vi "James_LED.vi"   [LabVIEW 2023]
uses:
  <vilib>/Rock Robotics/WPI/ThirdParty/PhotonVisionLib/PhotonVisionLib.lvlib
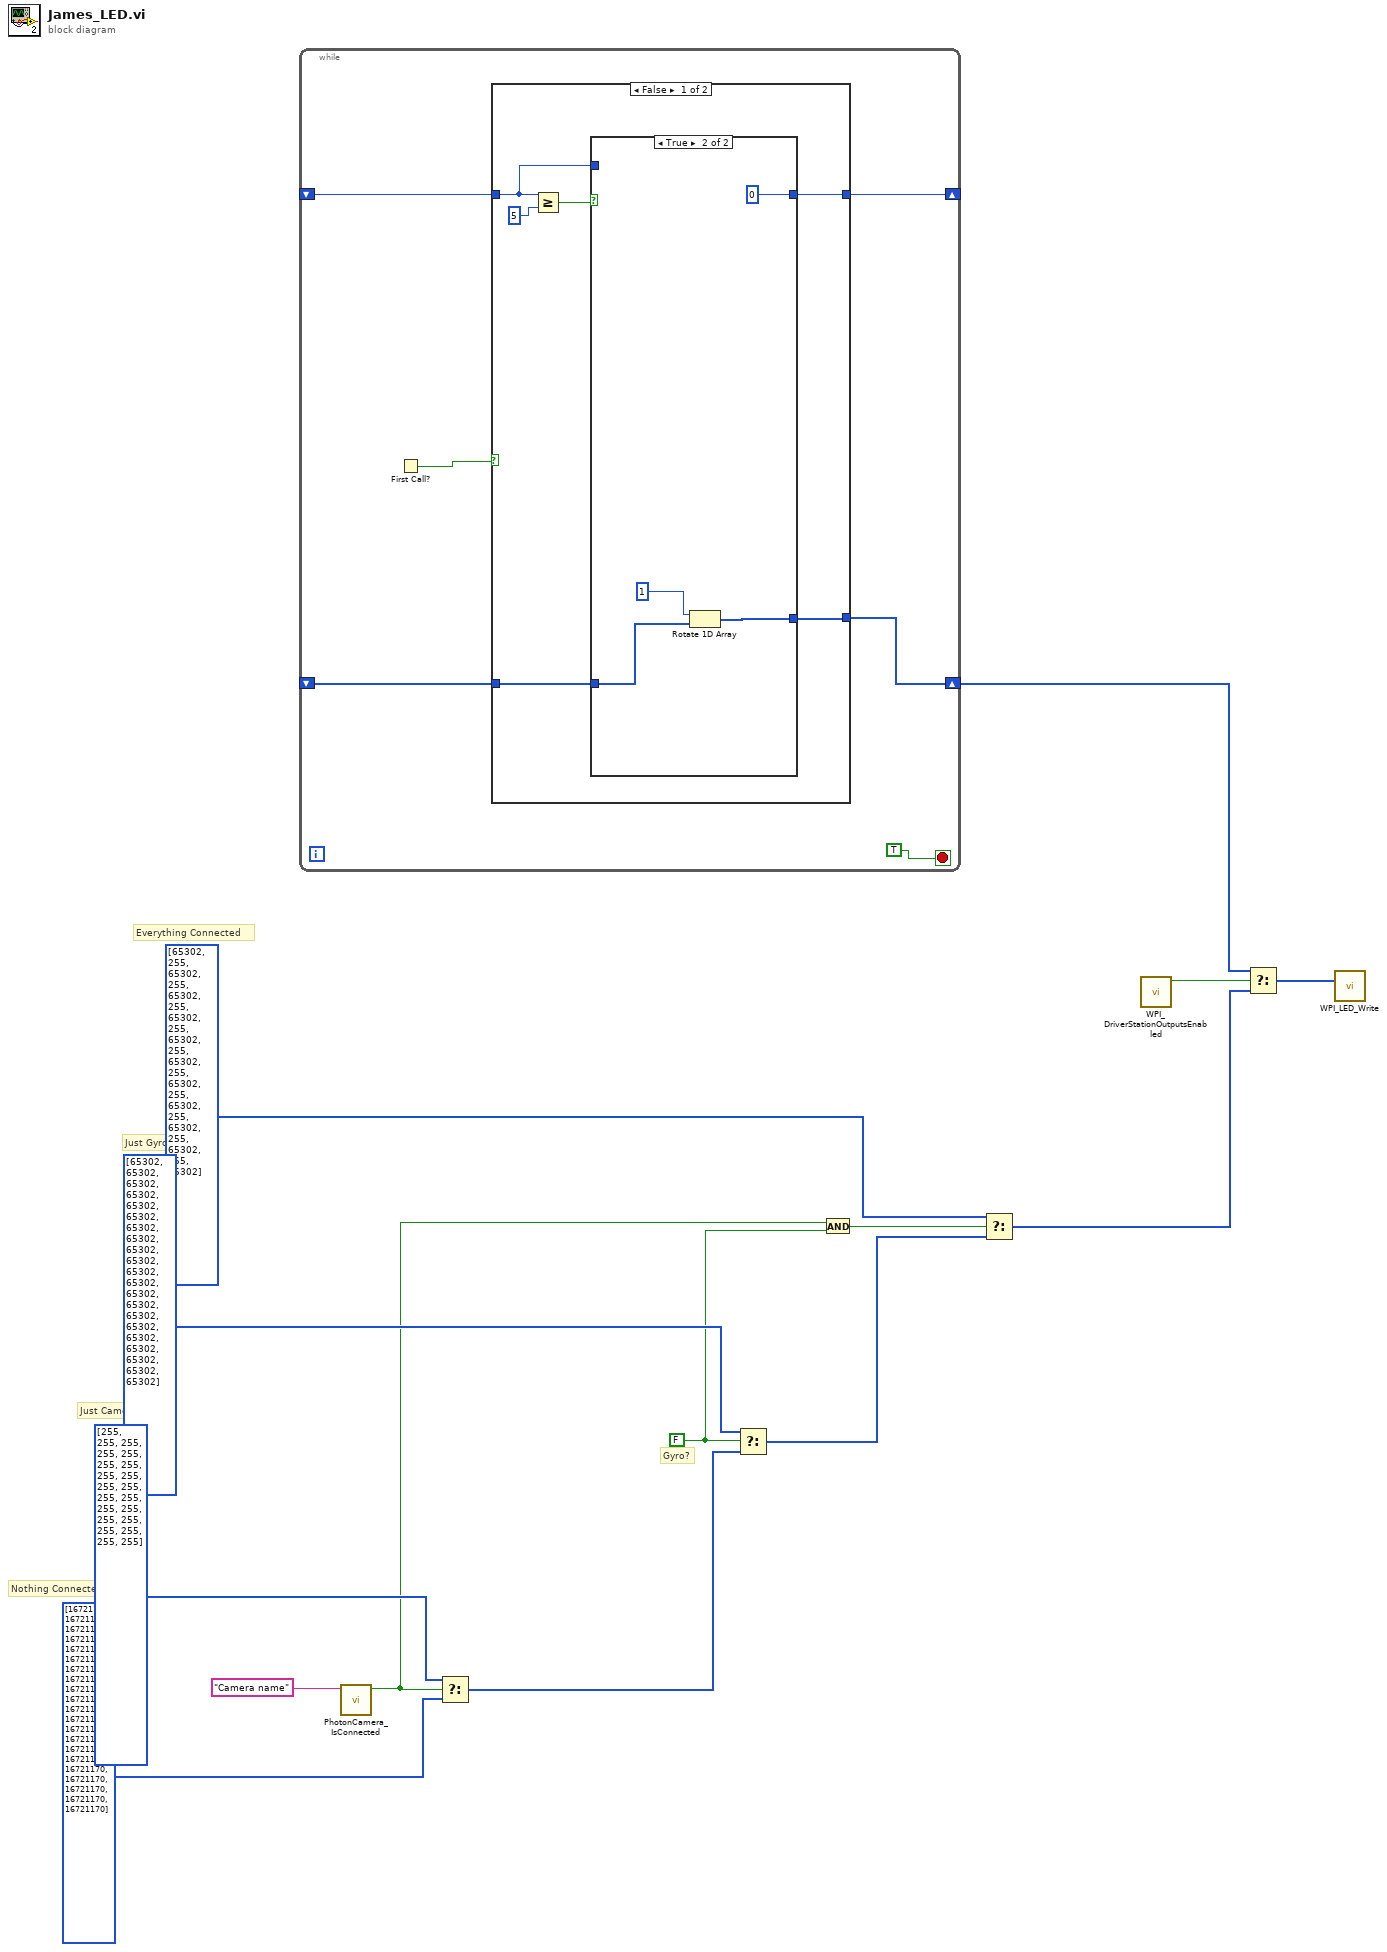
[diagram p0: block diagram]
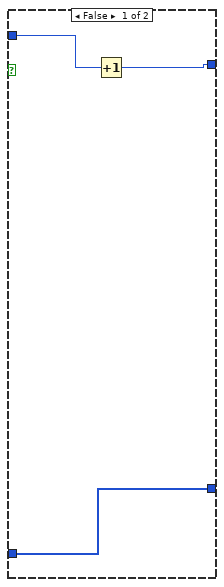
[diagram p2: hidden frame]
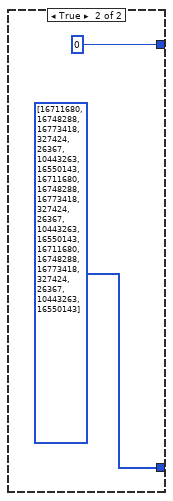
[diagram p3: hidden frame]
diagram:
  w7 = FALSE
  # "Gyro?"
  # "Everything Connected"
  # "Just Gyro"
  # "Just Camera"
  # "Nothing Connected"
  n1 = while {
    shift-right: [w18] -> w1
    shift-left: _ -> [w15]
    shift-right: [w17] -> _
    shift-left: _ -> [w16]
    stop <- TRUE stop-if-true
    n2 = First Call?() -> (First Call?: T/F=w19:bool)
    n3 = case shown="False" w19 {
      tunnel: [w23 u32[] [16711680, 16748288, 16773418, 327424, 26367, 10443263, 16550143, 16711680, 16748288, 16773418, 327424, 26367, 10443263, 16550143, 16711680, 16748288, 16773418, 327424, 26367, 10443263, 16550143] ("Color Array")] -> w18
      tunnel: [w22 0] -> w17
      tunnel: w16 -> [w21 _]
      tunnel: w15 -> [w24 _]
      frame False {
        n4 = Greater Or Equal?(x=w21, y=5) -> (x >= y?=w25:bool)
        n5 = case shown="True" w25 {
          tunnel: w24 -> [w27 w32]
          tunnel: [w27 w31] -> w23
          tunnel: [w29 0] -> w22
          tunnel: w21 -> [w28 _]
          frame False {
            n6 = Increment(x=w28) -> (x+1=w29:i32)
          }
          frame True {
            n7 = Rotate 1D Array(1:w32, 2:1 ("n")) -> (0:w31:u32[])
          }
        }
      }
      frame True {
      }
    }
  }
  n8 = call <vilib>:"PhotonCamera_IsConnected.vi"("CameraName"="Camera name") -> ("IsConnected"=w5:bool)  [unwired: 9 in, 1 out]
  n9 = Select(t=u32[] [255, 255, 255, 255, 255, 255, 255, 255, 255, 255, 255, 255, 255, 255, 255, 255, 255, 255, 255, 255, 255] ("Color Array"), s=w5, f=u32[] [16721170, 16721170, 16721170, 16721170, 16721170, 16721170, 16721170, 16721170, 16721170, 16721170, 16721170, 16721170, 16721170, 16721170, 16721170, 16721170, 16721170, 16721170, 16721170, 16721170, 16721170] ("Color Array")) -> (s? t:f=w14:u32[])
  n10 = Select(t=u32[] [65302, 65302, 65302, 65302, 65302, 65302, 65302, 65302, 65302, 65302, 65302, 65302, 65302, 65302, 65302, 65302, 65302, 65302, 65302, 65302, 65302] ("Color Array"), s=w7, f=w14) -> (s? t:f=w12:u32[])
  n11 = And(x=w5, y=w7) -> (x .and. y?=w11:bool)
  n12 = Select(t=u32[] [65302, 255, 65302, 255, 65302, 255, 65302, 255, 65302, 255, 65302, 255, 65302, 255, 65302, 255, 65302, 255, 65302, 255, 65302] ("Color Array"), s=w11, f=w12) -> (s? t:f=w3:u32[])
  n13 = call <vilib>:"WPI_DriverStationOutputsEnabled.vi"() -> ("OutputsEnabled?"=w4:bool)  [unwired: 10 in, 1 out]
  n14 = Select(t=w1, s=w4, f=w3) -> (s? t:f=w2:u32[])
  n15 = call <vilib>:"WPI_LED_Write.vi"("Color Array"=w2) -> ()  [unwired: 10 in, 1 out]
